vi "TMCM351-getAddress.vi"(2 "错误输入":errorcluster caption="错误输入（无错误）", 3 "com in":refnum<visa-resource-name>) -> (0 "错误输出":errorcluster, 1 "com out":refnum<visa-resource-name>)   [LabVIEW 2018]
uses:
  module_param.vi
panel:
  out "return out":u8[](array[numeric])
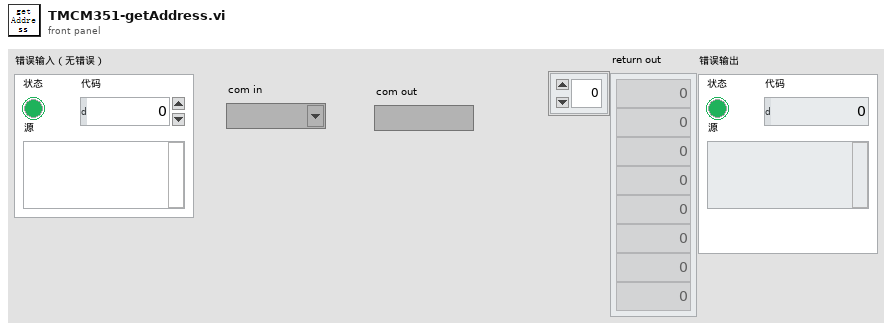
[diagram p1: front panel]
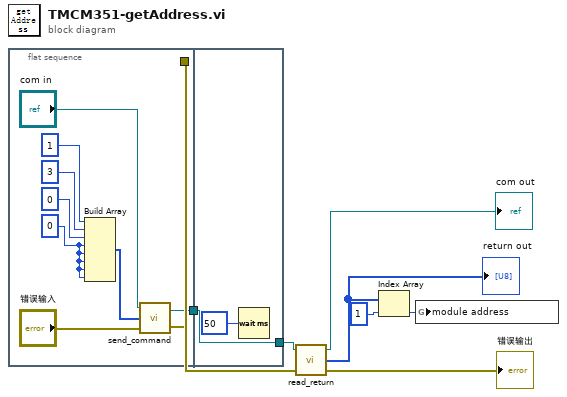
[diagram p0: block diagram]
diagram:
  n1 = flat-sequence {
    tunnel: [w12] -> w6
    tunnel: [w10] -> w5
    tunnel: [w19] -> w8
    tunnel: w6 -> [w19]
    frame #0 {
      w11 = u8 0 ("元素")
      n2 = Build Array(u8 1, u8 3, u8 0, w11, w11, w11, w11, w11) -> (w14:u8[])
      n3 = call "send_command.vi"("错误输入"="错误输入", 3:w14, "com in"="com in") -> ("错误输出"=w10:errorcluster, "com out"=w12:refnum<visa-resource-name>)
    }
    frame #1 {
      n4 = Wait (ms)(milliseconds to wait=u32 50 ("等待时间（毫秒）")) -> ()  [unwired: 1 out]
    }
  }
  n5 = call "read_return.vi"("错误输入（无错误）"=w5, "com in"=w8) -> ("错误输出"=→"错误输出":errorcluster, "return out"=w3:u8[], "com out"=→"com out":refnum<visa-resource-name>)  [unwired: 1 in]
  "return out" <- w3
  n6 = Index Array(array=w3, index=1 ("索引")) -> (element=w1:u8)
  n7 = global write "module_param.vi" "module address"(w1) -> ()
